vi "RunningAverage.vi"(11 "camtran (z)":dbl) -> (3 "mean":dbl format="%0.2f")   [LabVIEW 2019]
doc: "calculates the running average of a value"
uses:
  <vilib>/Analysis/baseanly.llb/Mean (DBL).vi
  <vilib>/Analysis/NI_AALBase.lvlib
panel:
  out "output array":dbl[](array[numeric])
  out "?":cluster{dbl, dbl}(graph)
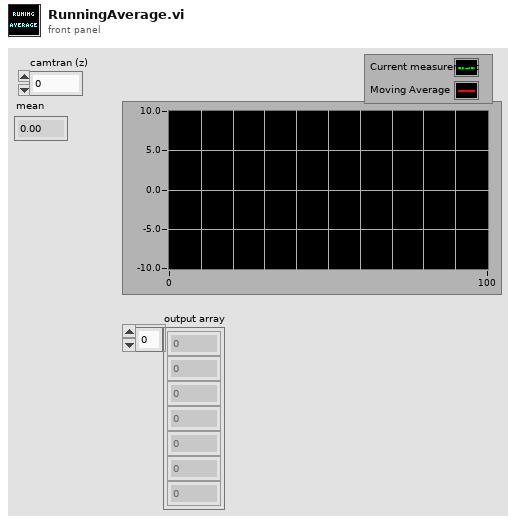
[diagram p1: front panel]
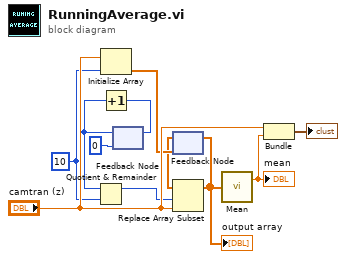
[diagram p0: block diagram]
diagram:
  w2 = 10 ("Average")
  n1 = Initialize Array("camtran (z)", w2) -> (w7:dbl[])
  n2 = feedback #1(0) -> (w10:i32)
  n3 = Quotient & Remainder(x=w10, y=w2) -> (x-y*floor(x/y)=w4:i32)  [unwired: 1 out]
  n4 = Increment(x=w10) -> (x+1=w9:i32)
  n5 = feedback-in #1(w9) -> ()
  n6 = feedback #2(w7) -> (w3:dbl[])
  n7 = Replace Array Subset(array=w3, new element="camtran (z)", index=w4) -> (w5:dbl[])
  "output array" <- w5
  n8 = feedback-in #2(w5) -> ()
  n9 = call-poly <vilib>:"Mean.vi"("X"=w5) -> ("mean"=w1:dbl)  [unwired: 1 out]
  "mean" <- w1
  n10 = Bundle("camtran (z)"="camtran (z)", "mean"=w1) -> (→"?":cluster{"camtran (z)":dbl, "mean":dbl})  [unwired: 1 in]
